vi "update_providers.vi"(8 "error in (no error)":errorcluster, 10 "log_entry":T1 {"datetime" format="%<%x %.3X>T"}, 11 "system.logging in":refnum<class "system.logging.lvclass">) -> (0 "error out":errorcluster, 3 "system.logging out":refnum<class "system.logging.lvclass">)   [LabVIEW 2021, in "system.logging.lvclass"]
uses:
  system.logging.lvclass
  log_entry.ctl
  severity.ctl
  system.logging.lvclass/system.logging.ctl
  system.logging.provider/system.logging.provider.lvclass
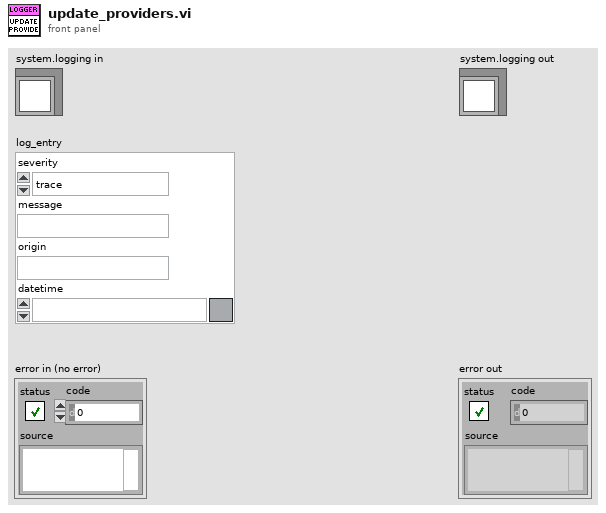
[diagram p1: front panel]
types:
  T1 = typedef "system.logging.lvclass/log_entry.ctl" = cluster{"severity":T2, "message":string, "origin":string, "datetime":timestamp}
  T2 = typedef "system.logging.lvclass/severity.ctl" = enum8{"trace", "debug", "info", "warning", "error"}
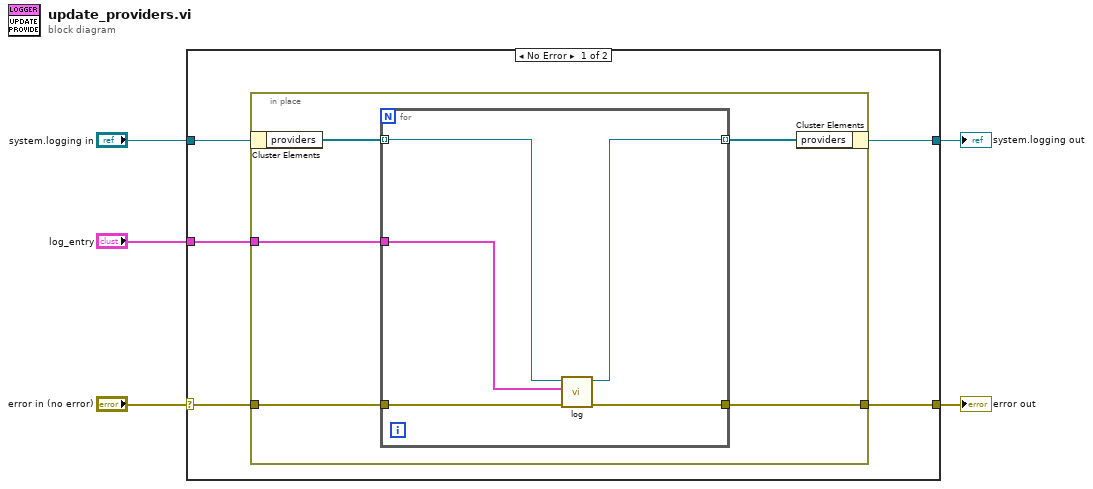
[diagram p0: block diagram]
diagram:
  n1 = case shown="No Error" "error in (no error)" {
    selector: "error in (no error)" -> [w8 w22]
    tunnel: [w7 w22] -> w4
    tunnel: [w6 w21] -> w2
    tunnel: "system.logging in" -> [w10 w21]
    tunnel: "log_entry" -> [w9 _]
    frame No Error {
      n2 = in-place {
        in-place-border: w9 -> [w14]
        in-place-border: w8 -> [w13]
        in-place-border: [w11] -> w7
        n3 = in-place-cluster #1(w10) -> ("providers"=w15:refnum<class "system.logging.provider.lvclass">[])
        n4 = for {
          tunnel: w15 -> [w18] mode=indexing
          tunnel: w14 -> [w19]
          tunnel: w13 -> [w20]
          tunnel: [w17] -> w12 mode=indexing
          tunnel: [w16] -> w11
          n5 = call-dynamic "log.vi"("error in (no error)"=w20, "log_entry"=w19, "system.logging.provider in"=w18) -> ("error out"=w16:errorcluster, "system.logging.provider out"=w17:refnum<class "system.logging.provider.lvclass">)  [unwired: 7 in]
        }
        n6 = in-place-cluster #1("providers"=w12) -> (w6:refnum<class "system.logging.lvclass">)
      }
    }
    frame Error {
    }
  }
  "error out" <- w4
  "system.logging out" <- w2
